vi "Files Change.vi"(8 "error in (no error)":errorcluster, 9 "Files old value":path[](array[path]), 10 "Files new value":path[](array[path]), 11 "XY WFRM Plot in":refnum<class "XY WFRM Plot.lvclass">) -> (0 "error out":errorcluster, 3 "XY WFRM Plot out":refnum<class "XY WFRM Plot.lvclass">)   [LabVIEW 2015, in "XY WFRM Plot.lvclass"]
uses:
  XY WFRM Plot.lvclass
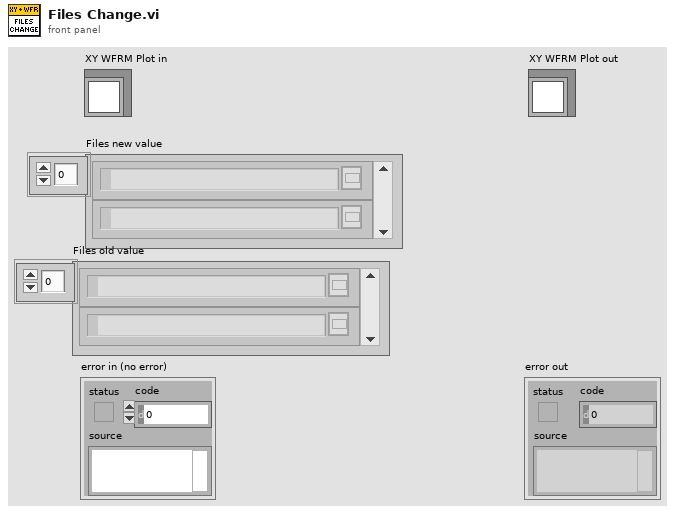
[diagram p1: front panel]
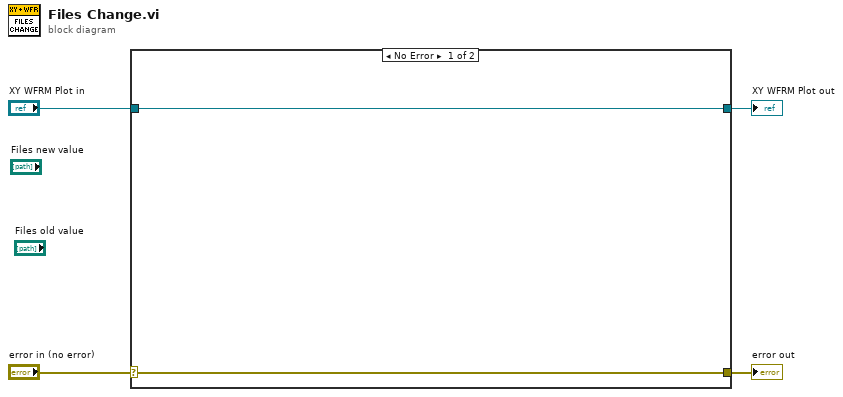
[diagram p0: block diagram]
diagram:
  n1 = case shown="No Error" "error in (no error)" {
    selector: "error in (no error)" -> [w5 w8]
    tunnel: [w5 w8] -> w3
    tunnel: [w6 w7] -> w1
    tunnel: "XY WFRM Plot in" -> [w6 w7]
    frame No Error {
    }
    frame Error {
    }
  }
  "error out" <- w3
  "XY WFRM Plot out" <- w1
